vi "Triangle Pattern.vi"(6 "asymmetry":dbl=0.5, 7 "width (s)":dbl=10.0, 8 "delta t (s)":dbl=0.1, 9 "delay (s)":dbl, 10 "amplitude":dbl=1.0, 11 "samples":i32=128) -> (0 "error":i32, 3 "Triangle Pattern":dbl[](array[numeric]))   [LabVIEW 2014, in "NI_AALBase.lvlib"]
doc: "Generates an array that contains a triangle pattern."
uses:
  NI_AALBase.lvlib
panel:
  # "Triangle Pattern"
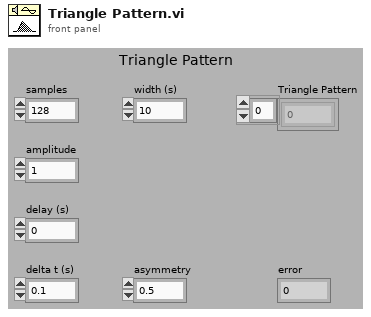
[diagram p1: front panel]
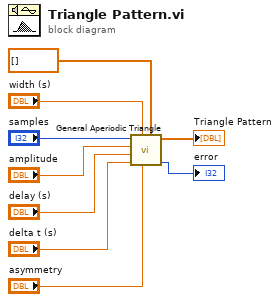
[diagram p0: block diagram]
diagram:
  n1 = call "General Aperiodic Triangle.vi"("X"=dbl[] [], "asymmetry"="asymmetry", "width"="width (s)", "delta t"="delta t (s)", "delay"="delay (s)", "amplitude"="amplitude", "samples"="samples") -> ("error"=→"error":i32, "Aperiod Triangle"=→"Triangle Pattern":dbl[])  [unwired: 3 in]
